vi "CONV String to 1D String.vi"(0 "String":string, 1 "Delimiter (,)":string=",") -> (6 "1-D String":string[](array[string]))   [LabVIEW 2017]
doc: "This routine converts a string list to a 1-D String array. String input may or may not have a trailing delimiter."
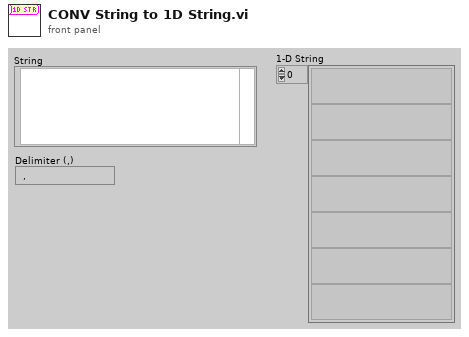
[diagram p1: front panel]
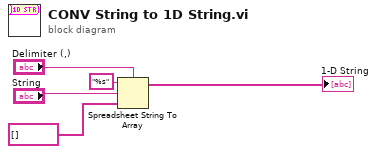
[diagram p0: block diagram]
diagram:
  n1 = Spreadsheet String To Array(delimiter (Tab)="Delimiter (,)", format string="%s", spreadsheet string="String", array type (2D Dbl)=string[] [] ("1-D String")) -> (array=→"1-D String":string[])
